vi "CRYCalc Eq Wave.vi"(9 "EQ Curve":T1={"Name"="", "Curve"=[], "X data"=1, "Y data"=1, "Z data"=1, "X axis"=0, "Y axis"=1, "Z axis"=1, "X unit"="Hz", "Y unit"="", "Z unit"="deg.", "X dB ref"=1.0, "Y dB ref"=1.0, "Z dB ref"=1.0, "single val"=FALSE, "protected"=FALSE, "display X"=TRUE, "display Y"=TRUE, "display Z"=TRUE, "Test Info"="", "Step No."=0, "Plot Settings"={"Color"=0, "Interpolation"=0, "Point Style"=0, "Line Style"=0, "Point Color"=0, "Line Width"=0, "Bar Plot Style"=0, "Fill To"=0}, "AutoProtect"=FALSE} {"Z data" items=["dB", "Lin"]; "X data" items=["dB", "Lin"]; "Y data" items=["dB", "Lin"]; "Z dB ref" format="%.1f"; "Z axis" items=["Log", "Lin"]; "X dB ref" format="%.1f"; "X axis" items=["Log", "Lin"]; "Y axis" items=["Log", "Lin"]; "Y dB ref" format="%.1f"; "Curve"."z" format="%.2f"; "Curve"."y" format="%.2f"; "Curve"."x" format="%.2f"}, 10 "Fs":dbl, 11 "Wave In":dbl[](array[numeric])) -> (2 "df":dbl, 3 "Wave Out":dbl[](array[numeric]))   [LabVIEW 2013]
uses:
  Typedef Control/CRYData Cluster.ctl
  <vilib>/Analysis/2dsp.llb/Real FFT.vi
  <vilib>/Analysis/2dsp.llb/Inverse Real FFT.vi
  <vilib>/Analysis/NI_AALPro.lvlib
panel:
  in  "Significant Digit":u8=2
  out "Waveform Graph 2":dbl[](graph)
  out "EQ":cluster{"x":dbl, "Lin Out":dbl}[](graph)
  out "Waveform Graph":dbl[](graph)
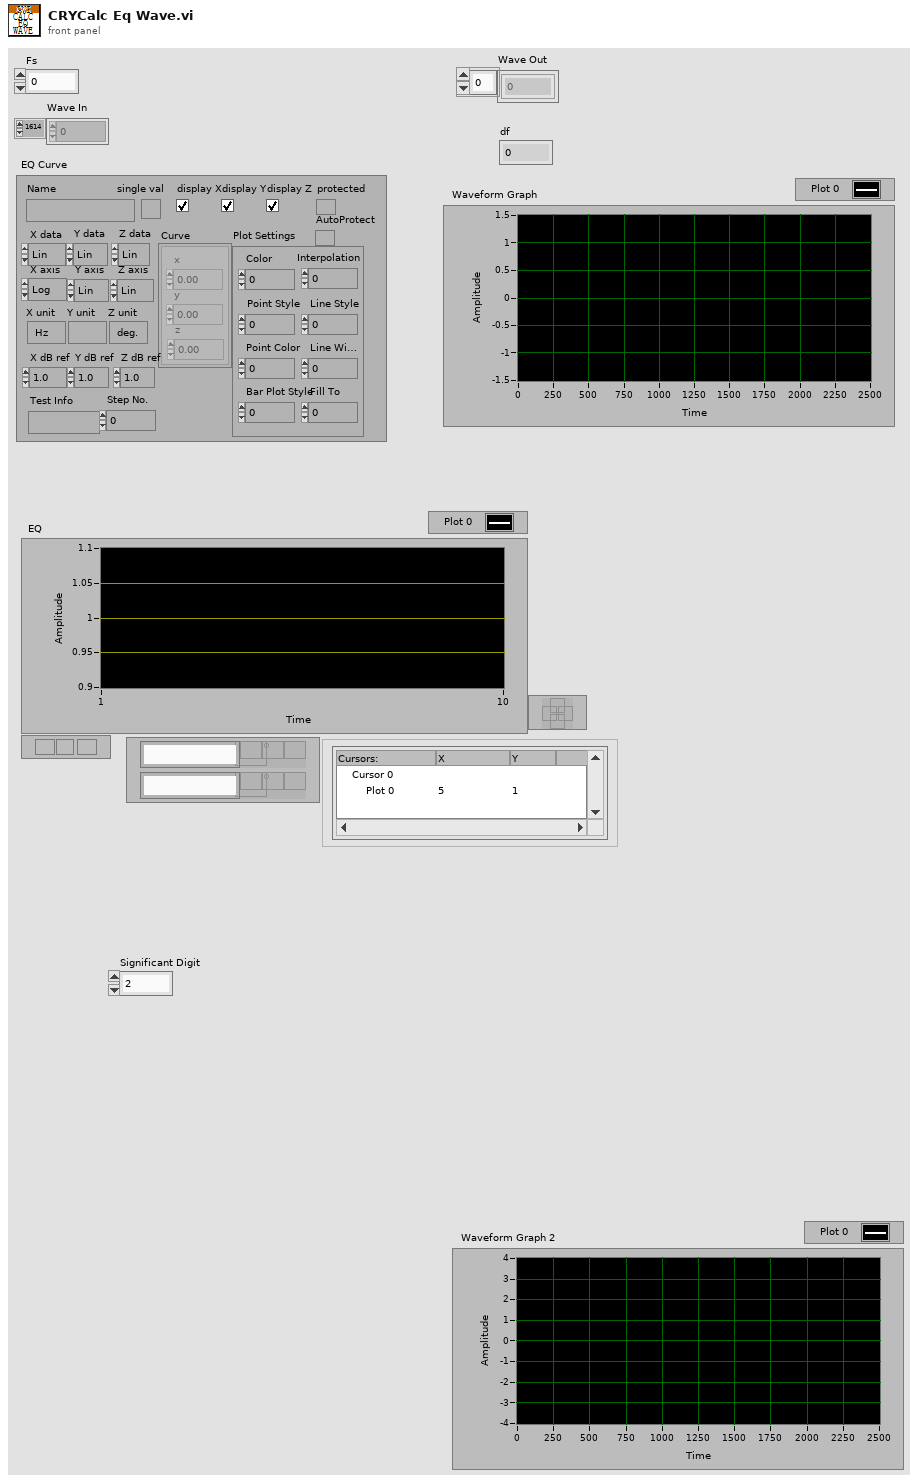
[diagram p1: front panel]
types:
  T1 = typedef "CRYData Cluster.ctl" = cluster{"Name":string, "Curve":cluster{"x":dbl, "y":dbl, "z":dbl}[], "X data":u16, "Y data":u16, "Z data":u16, "X axis":u16, "Y axis":u16, "Z axis":u16, "X unit":string, "Y unit":string, "Z unit":string, "X dB ref":dbl, "Y dB ref":dbl, "Z dB ref":dbl, "single val":bool, "protected":bool, "display X":bool, "display Y":bool, "display Z":bool, "Test Info":string, "Step No.":i32, "Plot Settings":cluster{"Color":u32, "Interpolation":u8, "Point Style":u8, "Line Style":u8, "Point Color":u32, "Line Width":u8, "Bar Plot Style":u8, "Fill To":i16}, "AutoProtect":bool}
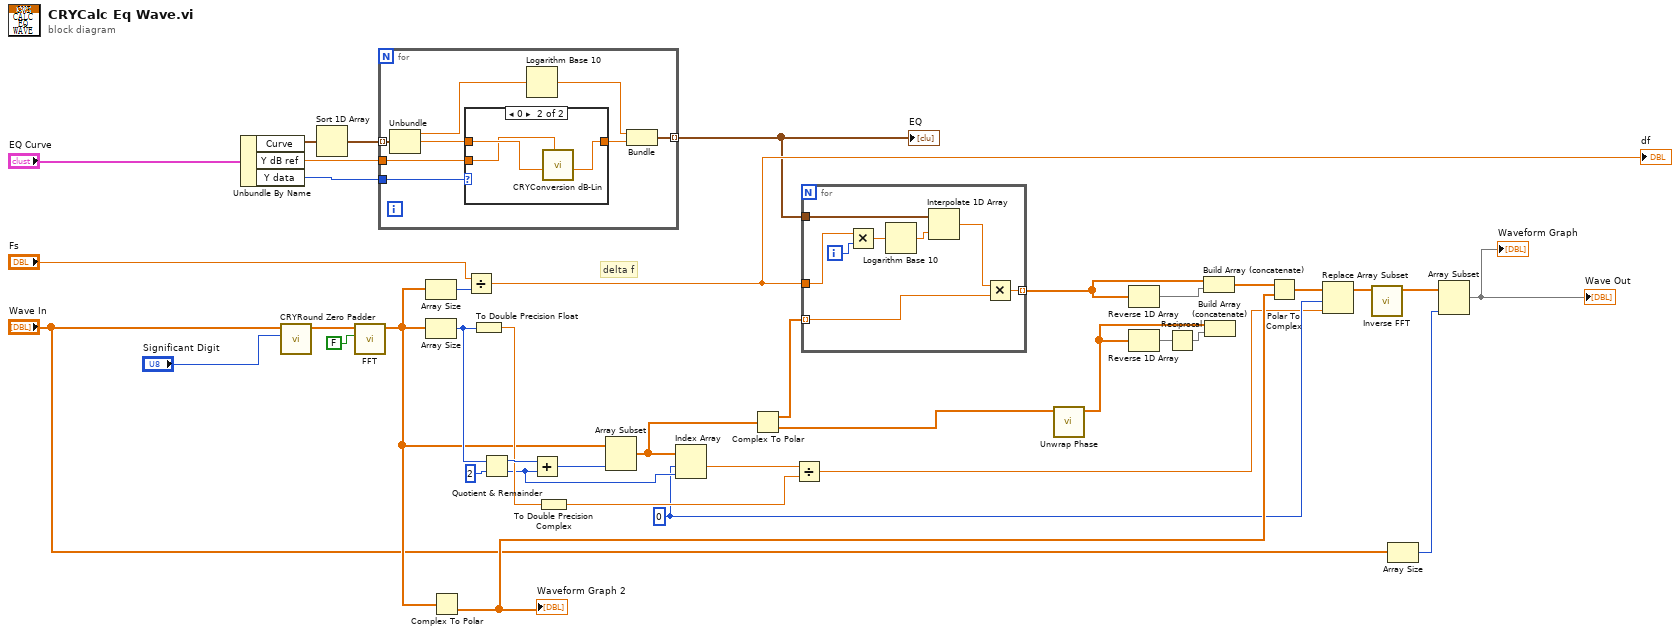
[diagram p0: block diagram]
diagram:
  w7 = 0 ("index")
  # "delta f"
  n1 = Unbundle By Name("EQ Curve") -> ("Curve"=w37:cluster{"x":dbl, "y":dbl, "z":dbl}[], "Y dB ref"=w36:dbl, "Y data"=w35:u16)
  n2 = call "CRYRound Zero Padder.vi"("Significant Digit"="Significant Digit", "Vector in"="Wave In") -> ("Zero Padder Vector out"=w2:dbl[])  [unwired: 8 in, 1 out]
  n3 = Sort 1D Array(array=w37) -> (sorted array=w10:cluster{"x":dbl, "y":dbl, "z":dbl}[])
  n4 = call-poly <vilib>:"FFT.vi"("shift?"=FALSE, "X"=w2) -> ("FFT {X}"=w17:cdb[])  [unwired: 8 in, 1 out]
  n5 = for {
    tunnel: w10 -> [w47] mode=indexing
    tunnel: [w46] -> w11 mode=indexing
    tunnel: w36 -> [w44]
    tunnel: w35 -> [w45]
    n6 = Unbundle(w47) -> ("x"=w41:dbl, "y"=w43:dbl)  [unwired: 1 out]
    n7 = case shown="0" w45 {
      tunnel: w43 -> [w48 w51]
      tunnel: [w48 w50] -> w42
      tunnel: w44 -> [_ w49]
      frame 1, Default {
      }
      frame 0 {
        n8 = call "CRYConversion dB-Lin.vi"("dB ref."=w49, "Log In"=w51) -> ("Lin Out"=w50:dbl)  [unwired: 4 in, 3 out]
      }
    }
    n9 = Logarithm Base 10(1:w41) -> (0:w40:dbl)
    n10 = Bundle(w40, "Lin Out"=w42) -> (w46:cluster{dbl, "Lin Out":dbl})  [unwired: 1 out]
  }
  "EQ" <- w11
  n11 = Array Size(array=w17) -> (size(s)=w34:i32)
  n12 = Array Size(array=w17) -> (size(s)=w28:i32)
  n13 = Complex To Polar(r * e^(i*theta)=w17) -> (theta=w14:dbl[])  [unwired: 1 out]
  "Waveform Graph 2" <- w14
  n14 = Divide(x="Fs", y=w34) -> (x/y=w24:dbl)
  "df" <- w24
  n15 = To Double Precision Float(number=w28) -> (double precision float=w27:dbl)
  n16 = Quotient & Remainder(x=w28, y=2) -> (x-y*floor(x/y)=w30:i32, floor(x/y)=w12:i32)
  n17 = Add(x=w30, y=w12) -> (x+y=w29:i32)
  n18 = To Double Precision Complex(1:w27) -> (0:w13:cdb)
  n19 = Array Subset(array=w17, length=w29) -> (w18:cdb[])  [unwired: 1 in]
  n20 = Index Array(array=w18, index #1=w7, index #2=w12) -> (element #1=w19:cdb)  [unwired: 1 out]
  n21 = Complex To Polar(r * e^(i*theta)=w18) -> (r=w26:dbl[], theta=w25:dbl[])
  n22 = Divide(x=w19, y=w13) -> (x/y=w6:cdb)
  n23 = for {
    tunnel: w26 -> [w55] mode=indexing
    tunnel: w11 -> [w59]
    tunnel: [w58] -> w9 mode=indexing
    tunnel: w24 -> [w57]
    i -> [w56]
    n24 = Multiply(x=w57, y=w56) -> (x*y=w54:dbl)
    n25 = Logarithm Base 10(1:w54) -> (0:w53:dbl)
    n26 = Interpolate 1D Array(1:w53, 2:w59) -> (0:w52:dbl)
    n27 = Multiply(x=w52, y=w55) -> (x*y=w58:dbl)
  }
  n28 = call <vilib>:"Unwrap Phase.vi"("Phase"=w25) -> ("Unwrapped Phase"=w21:dbl[])  [unwired: 9 in, 1 out]
  n29 = Reverse 1D Array(array=w9) -> (reversed array=w23:dbl[])
  n30 = Reverse 1D Array(array=w21) -> (reversed array=w16:dbl[])
  n31 = Reciprocal(x=w16) -> (1/x=w15:dbl[])
  n32 = Build Array (concatenate)(w9, w23) -> (w22:dbl[])
  n33 = Build Array (concatenate)(w21, w15) -> ()  [unwired: 1 out]
  n34 = Polar To Complex(1:w14, 2:w22) -> (0:w8:cdb[])
  n35 = Replace Array Subset(array=w8, new element=w6, index=w7) -> (w5:cdb[])
  n36 = call-poly <vilib>:"Inverse FFT.vi"("FFT {X}"=w5) -> ("X"=w32:dbl[])  [unwired: 9 in, 1 out]
  n37 = Array Size(array="Wave In") -> (size(s)=w33:i32)
  n38 = Array Subset(array=w32, length=w33) -> (→"Wave Out" →"Waveform Graph":dbl[])  [unwired: 1 in]
